vi "Main.vi"() -> ()   [LabVIEW 2015]
doc: "The myRIO Project template acquires acceleration data from the onboard accelerometer and displays the changes of acceleration values in a waveform chart."
uses:
  <vilib>/myRIO/Instrument Drivers/Onboard IO/DIO/typedefs/DIO Reference.ctl
  <vilib>/myRIO/Common/Instrument Driver Framework/Utilities/typedefs/myRIO Generic Hardware Reference.ctl
  <vilib>/myRIO/Common/Instrument Driver Framework/Utilities/typedefs/Hardware Version Enum.ctl
  <vilib>/myRIO/Common/Instrument Driver Framework/Utilities/typedefs/myRIO v1.0 Reference.ctl
  <vilib>/myRIO/Common/Instrument Driver Framework/Utilities/typedefs/Generic FPGA Reference.ctl
  <vilib>/myRIO/Common/Instrument Driver Framework/myRIO v1.0/DIO/typedefs/DIO Channels List.ctl
  <vilib>/myRIO/Common/Instrument Driver Framework/myRIO v1.0/DIO/typedefs/DIO Channels Enum.ctl
  <vilib>/userdefined/High Color/nirio_resource_hc.ctl
  <vilib>/myRIO/Common/Instrument Driver Framework/Utilities/vis/Is FPGA Ref Available.vi
  <vilib>/myRIO/Common/Instrument Driver Framework/myRIO v1.0/DIO/vis/myRIO v1.1 Open DIO.vi
  <vilib>/myRIO/Instrument Drivers/Onboard IO/DIO/vis/Read.vi
  <vilib>/myRIO/Instrument Drivers/Onboard IO/DIO/vis/Write.vi
  <vilib>/myRIO/Common/Instrument Driver Framework/Utilities/vis/Validate Channels.vi
  <vilib>/myRIO/Common/Instrument Driver Framework/myRIO v1.0/DIO/vis/myRIO v1.0 Reserve DIO.vi
  <vilib>/myRIO/Common/Instrument Driver Framework/myRIO v1.0/UART/vis/myRIO v1.0 Close UART.vi
  <vilib>/myRIO/Common/Instrument Driver Framework/myRIO v1.0/Resource Manager/vis/myRIO v1.0 Reserve Channel List.vi
  <vilib>/myRIO/Common/Instrument Driver Framework/myRIO v1.0/DIO/vis/myRIO v1.0 Build MUX Configuration DIO.vi
  <vilib>/myRIO/Common/Instrument Driver Framework/myRIO v1.0/Resource Manager/vis/myRIO v1.0 Reserve Channel.vi
  <vilib>/myRIO/Common/Instrument Driver Framework/myRIO v1.0/Resource Manager/vis/myRIO v1.0 Unreserve Channel.vi
  <vilib>/myRIO/Common/Instrument Driver Framework/myRIO v1.0/Resource Manager/vis/myRIO v1.0 Create Configuration List.vi
  <vilib>/myRIO/Common/Instrument Driver Framework/myRIO v1.0/Resource Manager/vis/myRIO v1.0 Build Mutex Name.vi
  <vilib>/Utility/VariantDataType/GetNumericInfo.vi
  <vilib>/Utility/error.llb/Error Cluster From Error Code.vi
  <vilib>/myRIO/Common/Instrument Driver Framework/myRIO v1.0/myRIO v1.1 Open.vi
  <vilib>/myRIO/Common/Instrument Driver Framework/Utilities/vis/IO Manager.vi
  <vilib>/myRIO/Common/Instrument Driver Framework/Utilities/vis/Configuration Manager.vi
  <vilib>/myRIO/Common/Instrument Driver Framework/myRIO v1.0/Resource Manager/vis/myRIO v1.0 Configure IO.vi
  <vilib>/myRIO/Common/Instrument Driver Framework/myRIO v1.0/myRIO v1.0 Close.vi
  <vilib>/myRIO/Common/Instrument Driver Framework/myRIO v1.0/DIO/vis/myRIO v1.0 Read DIO.vi
  <vilib>/myRIO/Common/Instrument Driver Framework/Utilities/vis/FPGA Ref Manager.vi
  <vilib>/myRIO/Common/Instrument Driver Framework/myRIO v1.0/myRIO v1.0 Reset FPGA.vi
  <vilib>/myRIO/Common/Instrument Driver Framework/myRIO v1.0/IRQ/vis/myRIO v1.0 IRQ Info FGV.vi
  <vilib>/myRIO/Common/Instrument Driver Framework/myRIO v1.0/IRQ/vis/myRIO v1.0 Timer IRQ Info FGV.vi
  <vilib>/myRIO/Common/Instrument Driver Framework/myRIO v1.0/IRQ/vis/myRIO v1.0 ISR Agent.vi
  <vilib>/myRIO/Common/Instrument Driver Framework/myRIO v1.0/DIO/vis/myRIO v1.0 Write DIO.vi
  <vilib>/myRIO/Express VI/Onboard Devices/Button/Button Express VI.xnode
  <vilib>/myRIO/Instrument Drivers/Onboard IO/DIO/vis/myRIO DIO Open.xnode
  <vilib>/myRIO/Express VI/Onboard Devices/LED/LED Express VI.xnode
  <vilib>/myRIO/Instrument Drivers/Onboard IO/DIO/DIO.lvlib
  <vilib>/myRIO/Instrument Drivers/Utilities/Utilities.lvlib
panel:
  out "output cluster":T1 {"Numeric Control 2" format="%.2f"}
  in  "Stop":bool
  out "Saved file to path":path
  # "Timestamp"
  # "Temperature Value"
  # "Measured Resistance"
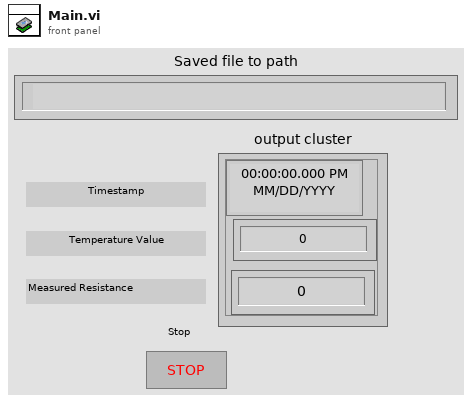
[diagram p1: front panel]
types:
  T1 = cluster{timestamp, "Numeric Control":dbl, "Numeric Control 2":u32}
  T2 = enum16{"open", "replace", "create", "open or create", "replace or create", "replace or create with confirmation"}
  T3 = typedef "DIO.lvlib/DIO Reference.ctl" = cluster{"myRIO Reference":T4, "DIO Channels List":T8}
  T4 = typedef "myRIO Generic Hardware Reference.ctl" = cluster{"myRIO Model":T5, "myRIO Hardware Reference":T6}
  T5 = typedef "Hardware Version Enum.ctl" = enum16{"Unknown", "myRIO-1900", "myRIO-1950", "roboRIO"}
  T6 = typedef "myRIO v1.0 Reference.ctl" = cluster{"Generic FPGA Reference":T7, "Allow multiple opens":bool}
  T7 = typedef "Generic FPGA Reference.ctl" = refnum<k20>
  T8 = typedef "DIO Channels List.ctl" = T9[]
  T9 = typedef "DIO Channels Enum.ctl" = enum16{"Not Connected", "C/DIO0", "C/DIO1", "C/DIO2", "C/DIO3", "C/DIO4", "C/DIO5", "C/DIO6", "C/DIO7", "A/DIO0", "A/DIO1", "A/DIO2", "A/DIO3", "A/DIO4", "A/DIO5", "A/DIO6", "A/DIO7", "A/DIO8", "A/DIO9", "A/DIO10", "A/DIO11", "A/DIO12", "A/DIO13", "A/DIO14", "A/DIO15", "B/DIO0", "B/DIO1", "B/DIO2", "B/DIO3", "B/DIO4", "B/DIO5", "B/DIO6", "B/DIO7", "B/DIO8", "B/DIO9", "B/DIO10", "B/DIO11", "B/DIO12", "B/DIO13", "B/DIO14", "B/DIO15", "LED0", "LED1", "LED2", "LED3", "Button0", "DIO/DIO0", "DIO/DIO1", "DIO/DIO2", "DIO/DIO3", "DIO/DIO4", "DIO/DIO5", "DIO/DIO6", "DIO/DIO7", "DIO/DIO8", "DIO/DIO9", "SPI/CS0", "SPI/CS1", "SPI/CS2", "SPI/CS3", "LED RADIO (Green)", "LED RADIO (Red)", "LED COMM (Green)", "LED COMM (Red)", "LED MODE (Green)", "LED MODE (Red)"}
  T10 = typedef "nirio_resource_hc.ctl" = tag
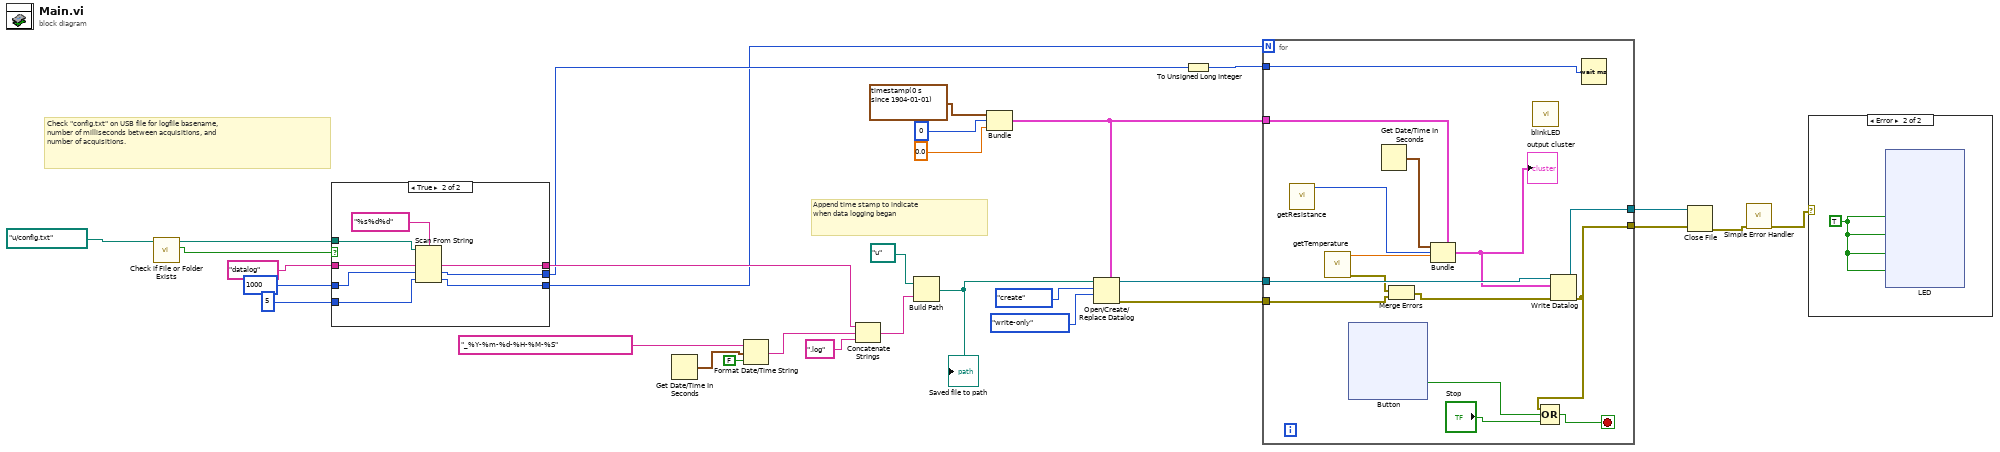
[diagram p0: block diagram]
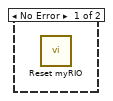
[diagram p2: hidden frame]
diagram:
  # "Append time stamp to indicate\nwhen data logging began"
  # "Check \"config.txt\" on USB file for logfile basename,\nnumber of milliseconds between acquisitions, and\nnumber of acquisitions."
  n1 = call <vilib>:"Check if File or Folder Exists.vi"("path"=path "u:/config.txt") -> ("file or folder exists?"=w29:bool, "dup path"=w28:path)  [unwired: 8 in, 1 out]
  n2 = case shown="True" w29 {
    tunnel: w28 -> [_ w41]
    tunnel: 5 ("default value 3") -> [w32 w40]
    tunnel: 1000 ("default value 2") -> [w31 w39]
    tunnel: "datalog" ("default value 1") -> [w33 w38]
    tunnel: [w33 w36] -> w22
    tunnel: [w31 w35] -> w12
    tunnel: [w32 w34] -> w11
    frame False {
    }
    frame True {
      n3 = Scan From String("%s%d%d" ("format string"), w41, default 1=w38, default 2=w39, default 3=w40) -> (output 1=w36:string, output 2=w35:i32, output 3=w34:i32)  [unwired: 1 in, 2 out]
    }
  }
  n4 = Get Date/Time In Seconds() -> (seconds since 1Jan1904=w1:timestamp)
  n5 = Format Date/Time String(time format string (%c)="_%Y-%m-%d-%H-%M-%S", seconds (now)=w1, UTC format=FALSE) -> (date/time string=w23:string)
  n6 = Concatenate Strings(w22, w23, ".log" ("string")) -> (w20:string)
  n7 = Build Path(base path=path "u:/", name or relative path=w20) -> (appended path=w16:path)
  "Saved file to path" <- w16
  n8 = Bundle(timestamp(0 s since 1904-01-01), u32 0, 0.0) -> (w7:cluster{timestamp, u32, dbl})  [unwired: 1 in]
  n9 = Open/Create/Replace Datalog(5:w7, 9:enum16{"read/write", "read-only", "write-only"}."write-only" ("access (0:read/write)"), 10:T2."create" ("operation (0:open)"), 11:w16) -> (0:w8:errorcluster, 3:w9:refnum<k1>)  [unwired: 2 in, 1 out]
  n10 = To Unsigned Long Integer(number=w12) -> (unsigned 32bit integer=w13:u32)
  n11 = for {
    N: w11 -> [_]
    tunnel: w13 -> [w53]
    tunnel: w9 -> [w51]
    tunnel: w8 -> [w44]
    tunnel: [w52] -> w6
    tunnel: w7 -> [w49]
    tunnel: [w47] -> w4
    stop <- w56 stop-if-true
    n12 = call "getResistance.vi"() -> ("Measured Resistance"=w46:u32)  [unwired: 11 in]
    n13 = call "getTemperature.vi"() -> ("error out"=w43:errorcluster, "Measured Temperature [*C]"=w45:dbl)  [unwired: 10 in]
    n14 = xnode "Button"() -> ("Value"=w54:bool)  [unwired: 1 in, 1 out]
    n15 = Get Date/Time In Seconds() -> (seconds since 1Jan1904=w48:timestamp)
    n16 = Merge Errors(w43, w44) -> (w42:errorcluster)
    n17 = Bundle(cluster=w49, w48, w46, w45) -> (w50:cluster{timestamp, u32, dbl})
    "output cluster" <- w50
    n18 = call "blinkLED.vi"() -> ()  [unwired: 12 in]
    n19 = Write Datalog(4:w42, 6:w50, 7:w51) -> (0:w52:errorcluster, 3:w47:refnum<k1>)
    n20 = Compound Arithmetic op=OR(w52, w54, "Stop") -> (w56:bool)
    n21 = Wait (ms)(milliseconds to wait=w53) -> ()  [unwired: 1 out]
  }
  n22 = Close File(refnum=w4, error in=w6) -> (error out=w5:errorcluster)  [unwired: 1 out]
  n23 = call <vilib>:"Simple Error Handler.vi"("error in (no error)"=w5) -> ("error out"=w10:errorcluster)  [unwired: 4 in, 4 out]
  n24 = case shown="Error" w10 {
    frame No Error {
      n25 = call <vilib>:"Reset myRIO.vi"() -> ()  [unwired: 11 in, 1 out]
    }
    frame Error {
      w92 = TRUE
      n26 = xnode "LED"("LED0"=w92, "LED1"=w92, "LED2"=w92, "LED3"=w92) -> ()  [unwired: 1 in, 1 out]
    }
  }
